vi "Reset Front Panel.vi"(11 "output cluster":T1) -> (0 "error out":errorcluster)   [LabVIEW 2022 SP3]
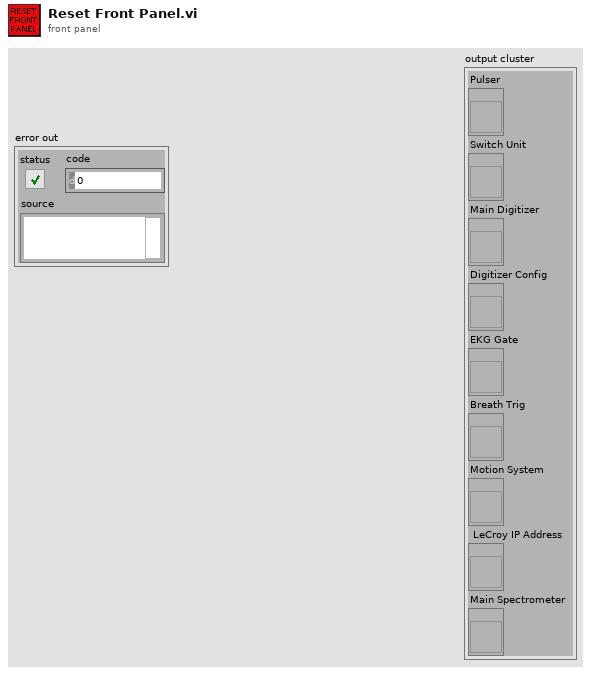
[diagram p1: front panel]
types:
  T1 = cluster{"Pulser":refnum<vi>, "Switch Unit":refnum<vi>, "Main Digitizer":refnum<vi>, "Digitizer Config":refnum<vi>, "EKG Gate":refnum<vi>, "Breath Trig":refnum<vi>, "Motion System":refnum<vi>, " LeCroy IP Address":refnum<vi>, "Main Spectrometer":refnum<vi>}
  T2 = enum8{"Enabled", "Disabled", "Disabled and Grayed Out"}
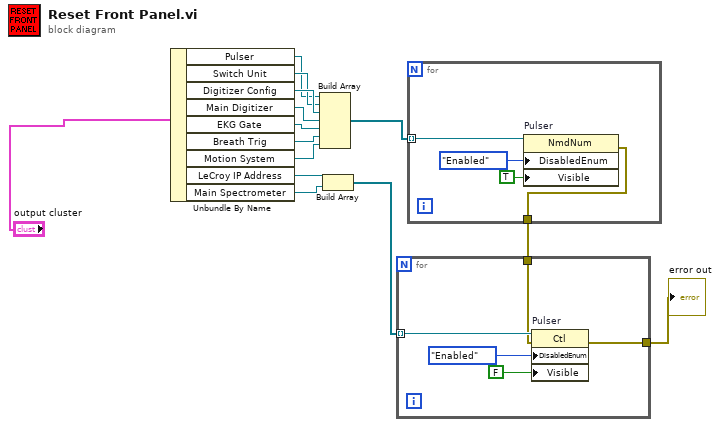
[diagram p0: block diagram]
diagram:
  n1 = Unbundle By Name("output cluster") -> ("Pulser"=w2:refnum<vi>, "Switch Unit"=w3:refnum<vi>, "Digitizer Config"=w4:refnum<vi>, "Main Digitizer"=w5:refnum<vi>, "EKG Gate"=w6:refnum<vi>, "Breath Trig"=w7:refnum<vi>, "Motion System"=w8:refnum<vi>, "LeCroy IP Address"=w10:refnum<vi>, "Main Spectrometer"=w11:refnum<vi>)
  n2 = Build Array(w2, w3, w4, w5, w6, w7, w8) -> (w9:refnum<vi>[])
  n3 = Build Array(w10, w11) -> (w12:refnum<vi>[])
  n4 = for {
    tunnel: w9 -> [w17] mode=indexing
    tunnel: [w15] -> w13
    n5 = property on="Pulser" class="NmdNum"(reference=w17, "DisabledEnum"=T2."Enabled" ("Disabled"), "Visible"=TRUE) -> (error out=w15:errorcluster)  [unwired: 1 in, 1 out]
  }
  n6 = for {
    tunnel: w12 -> [w22] mode=indexing
    tunnel: w13 -> [w20]
    tunnel: [w19] -> w14
    n7 = property on="Pulser" class="Ctl"(reference=w22, error in=w20, "DisabledEnum"=T2."Enabled" ("Disabled"), "Visible"=FALSE) -> (error out=w19:errorcluster)  [unwired: 1 out]
  }
  "error out" <- w14
